vi "HEWH RLT Cutout Checker.vi"(0 "Station":string, 2 "Current (Amps)":dbl, 3 "Delay After Cutout (sec)":dbl, 5 "error in (no error)":errorcluster, 8 "Use Cutout Delay":bool, 9 "Start Draw":bool, 10 "Station Data Input":T2={"Sequence #"=0.0, "Cycles"=0, "Mode Setting"="", "Flow Rate (GPM)"=0.0, "Temperature (F)"=0.0, "Reset Timer"=FALSE, "Use Temp Decline Method"=FALSE, "Terminate Condition"=enum."C1-Terminate Draw @ Gallon Mark", "Condition Value #1"=0.0, "UE"=FALSE, "LE"=FALSE, "Comp"=FALSE, "Fan"=FALSE, "Test End Time (Sec)"=0.0, "Purge Until Cutout"=FALSE, "Start Conditions"=enum."Heat Source Cutout", "Condition Value #2"=0.0, "Remove Power"=FALSE, "Time"=0.0, "Check Special Cond."=enum."SC2-Check Heat Source (On-C2/Off-C1)", "Condition#"=enum."C1", "Draw Flags"=enum."N/A", "Data Processing Delay (FHD 15sec, UEF 5 Sec)"=0.0, "Test Complete"=FALSE} {"Time" format="%<%H:%M:%S>t"}, 11 "Debug Events":T1, 13 "Debug":bool) -> (14 "Full Cutout?":bool, 19 "error out":errorcluster)   [LabVIEW 2016]
uses:
  Type Definitions/PRAT Test.ctl
  Utility/Save File/File Setup (Public)/Type Definition/Save File HEWH Heating Control Mode.ctl
  Draw Water Specific/Type Definitions/Terminate Draw Conditions.ctl
  Type Definitions/HEWH Start Conditions.ctl
  Draw Water Specific/Type Definitions/Check Special Condtions.ctl
  Draw Water Specific/Type Definitions/HEWH Special Condition Check.ctl
  Type Definitions/HEWH Draw Flag ENUM.ctl
  Type Definitions/HEWH Power Elements.ctl
  Utility/Type Definitions/UTILITY Notifier.ctl
  Utility/Save File/File Setup.lvlib
panel:
  out "Array":bool[](array[boolean])
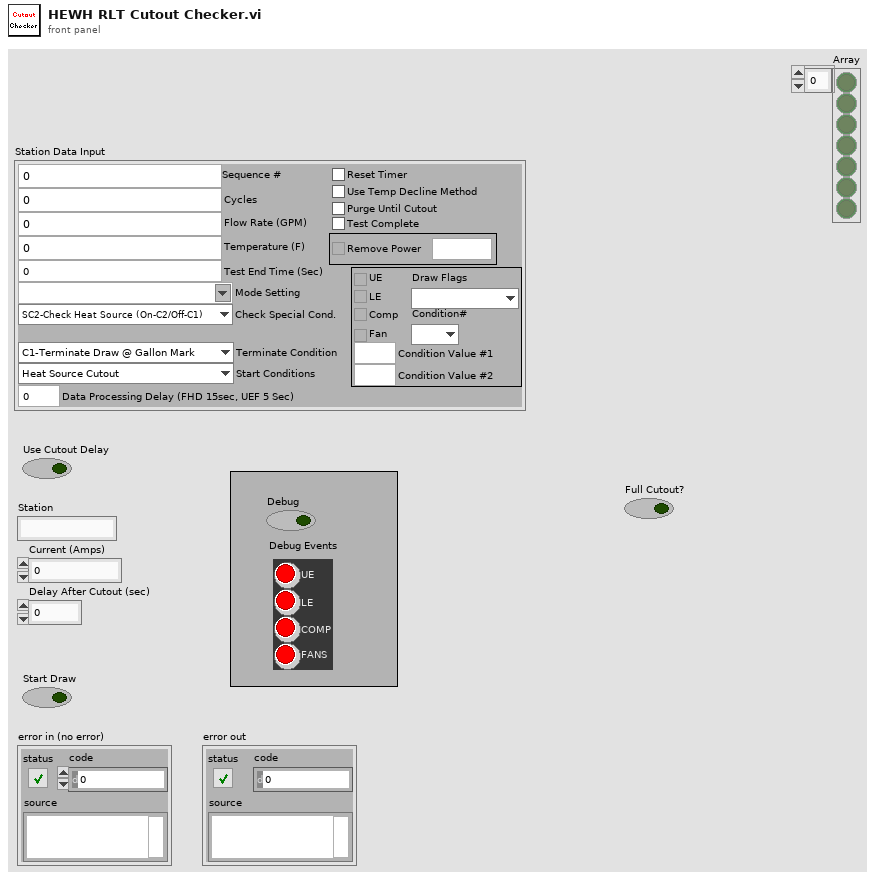
[diagram p1: front panel]
types:
  T1 = typedef "HEWH Power Elements.ctl" = cluster{"UE":bool, "LE":bool, "COMP":bool, "FANS":bool}
  T2 = typedef "PRAT Test.ctl" = cluster{"Sequence #":dbl, "Cycles":i32, "Mode Setting":T3, "Flow Rate (GPM)":dbl, "Temperature (F)":dbl, "Reset Timer":bool, "Use Temp Decline Method":bool, "Terminate Condition":T4, "Condition Value #1":dbl, "UE":bool, "LE":bool, "Comp":bool, "Fan":bool, "Test End Time (Sec)":dbl, "Purge Until Cutout":bool, "Start Conditions":T5, "Condition Value #2":dbl, "Remove Power":bool, "Time":dbl, "Check Special Cond.":T6, "Condition#":T7, "Draw Flags":T8, "Data Processing Delay (FHD 15sec, UEF 5 Sec)":dbl, "Test Complete":bool}
  T3 = typedef "File Setup.lvlib/Save File HEWH Heating Control Mode.ctl" = string
  T4 = typedef "Terminate Draw Conditions.ctl" = enum16{"C1-Terminate Draw @ Gallon Mark", "C2-Special Last Draw (HU Test)", "C3-RTD Out <=", "C4-Mean Tank Temp <=", "C5-Decrease RTD Out (Deg F)", "C6-Time (Seconds)", "C7-Until Any Heat Source", "C8-Specific Heat Source", "C9-Do Nothing"}
  T5 = typedef "HEWH Start Conditions.ctl" = enum16{"Heat Source Cutout", "At Time (Seconds)", "Every X (Seconds)", "T2 >= X° Below Setpoint", "Seconds From Complete", "Wait for LE & Comp Cutout", "Wait for Comp Cutout", "Wait for LE Cutout", "Wait for UE Cutout"}
  T6 = typedef "Check Special Condtions.ctl" = enum16{"SC1-Do Nothing", "SC2-Check Heat Source (On-C2/Off-C1)", "SC3-Check Skip Condition", "SC4-Check Heat Source ON/Fail"}
  T7 = typedef "HEWH Special Condition Check.ctl" = enum16{"N/A", "C1", "C2", "Reset/Fail", "Skip Draw Sequence"}
  T8 = typedef "HEWH Draw Flag ENUM.ctl" = enum16{"N/A", "None(0)", "Sml(1)", "Med(2)", "SmlMed(3)", "Lrg(4)", "SmlLrg(5)", "MedLrg(6)", "SmlMedLrg(7)"}
  T9 = typedef "UTILITY Notifier.ctl" = enum16{"Set", "Read", "Release Ref"}
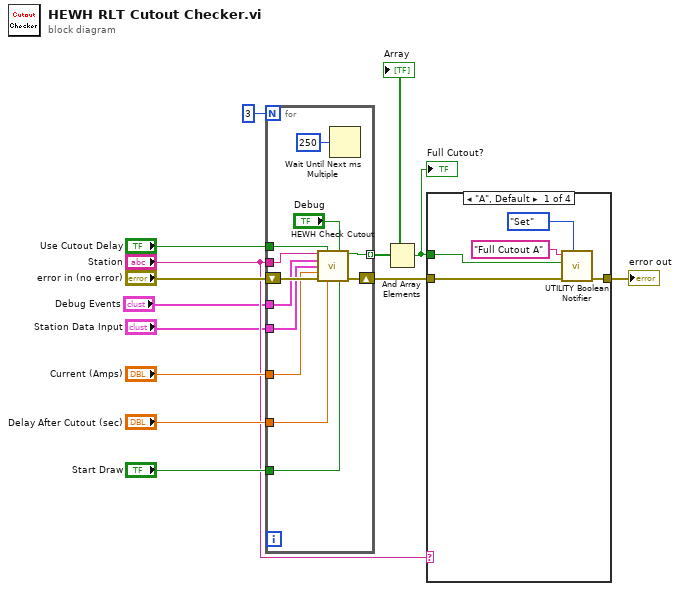
[diagram p0: block diagram]
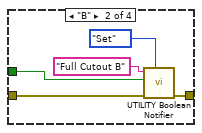
[diagram p2: hidden frame]
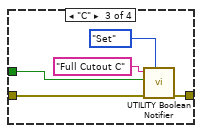
[diagram p3: hidden frame]
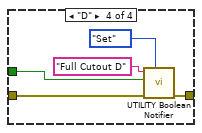
[diagram p4: hidden frame]
diagram:
  n1 = for {
    N: 3 -> [_]
    tunnel: [w25] -> w8 mode=indexing
    tunnel: "Station" -> [w24]
    shift-right: [w22] -> w4
    shift-left: "error in (no error)" -> [w23]
    tunnel: "Delay After Cutout (sec)" -> [w21]
    tunnel: "Use Cutout Delay" -> [w20]
    tunnel: "Current (Amps)" -> [w19]
    tunnel: "Start Draw" -> [w18]
    tunnel: "Station Data Input" -> [w16]
    tunnel: "Debug Events" -> [w14]
    n2 = call "HEWH Check Cutout.vi"("Station"=w24, "Use Cutout Delay"=w20, "Debug"="Debug", "Debug Events"=w14, "Station Data Input"=w16, "Current (Amps)"=w19, "Error In"=w23, "Delay After Cutout (sec)"=w21, "Start Draw"=w18) -> ("Full Cutout?"=w25:bool, "Error Out"=w22:errorcluster)  [unwired: 5 in]
    n3 = Wait Until Next ms Multiple(millisecond multiple=u32 250) -> ()  [unwired: 1 out]
  }
  "Array" <- w8
  n4 = And Array Elements(Boolean array=w8) -> (logical AND=w6:bool)
  "Full Cutout?" <- w6
  n5 = case shown="\"A\", Default" "Station" {
    tunnel: w6 -> [w28 w31 w36 w41]
    tunnel: [w27 w32 w37 w42] -> w5
    tunnel: w4 -> [w26 w33 w38 w43]
    frame "A", Default {
      n6 = call "UTILITY Boolean Notifier.vi"("Status"=UTILITY_Notifier."Set", "error in (no error)"=w26, "Set Status"=w28, "name (unnamed)"="Full Cutout A") -> ("error out"=w27:errorcluster)  [unwired: 6 in, 1 out]
    }
    frame "B" {
      n7 = call "UTILITY Boolean Notifier.vi"("Status"=UTILITY_Notifier."Set", "error in (no error)"=w33, "Set Status"=w31, "name (unnamed)"="Full Cutout B") -> ("error out"=w32:errorcluster)  [unwired: 6 in, 1 out]
    }
    frame "C" {
      n8 = call "UTILITY Boolean Notifier.vi"("Status"=UTILITY_Notifier."Set", "error in (no error)"=w38, "Set Status"=w36, "name (unnamed)"="Full Cutout C") -> ("error out"=w37:errorcluster)  [unwired: 6 in, 1 out]
    }
    frame "D" {
      n9 = call "UTILITY Boolean Notifier.vi"("Status"=UTILITY_Notifier."Set", "error in (no error)"=w43, "Set Status"=w41, "name (unnamed)"="Full Cutout D") -> ("error out"=w42:errorcluster)  [unwired: 6 in, 1 out]
    }
  }
  "error out" <- w5
